vi "StartAll.vi"(8 "Error In":errorcluster[](array[cluster])) -> (0 "Error Out":errorcluster[](array[cluster]), 2 "BC_AppInfo":T1)   [LabVIEW 2014, in "BusController.lvlib"]
uses:
  BusController.lvlib
  Modules/AppModule/PublicAPI/Arguments/Requests/BC_AppInfo.ctl
  Admin/Registry/BCReg.lvclass
  Queue/QueueType.ctl
  Admin/BCAdmin.lvclass/BCAdmin.ctl
  Admin/Accessors/Read BCRegRef.vi
  BusController.vi
  Bus_class/Bus.lvclass
  Framework.lvlib
  <userlib>/NIST/NISTErrorLib/NISTErrorLib.lvlib
  Modules/AppModule/AppModule.lvlib
  Admin/BCAdmin.lvclass
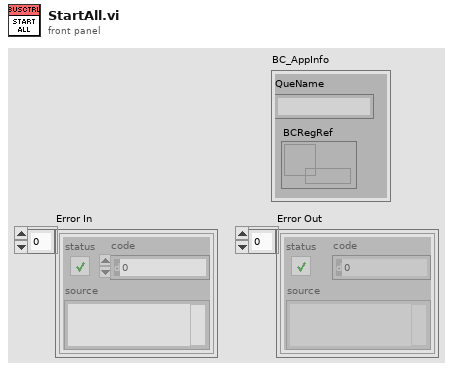
[diagram p1: front panel]
types:
  T1 = typedef "AppModule.lvlib/BC_AppInfo.ctl" = cluster{"QueName":string, "BCRegRef":refnum<data-value>}
  T2 = typedef "BusController.lvlib/QueueType.ctl" = cluster{"Msg":string, "Data":variant}
  T3 = typedef "Framework.lvlib/clFrameworkData.ctl" = cluster{"EvtINIFilePaths":path[], "BusClassInstances":refnum<class "Bus.lvclass">[], "PmuImpairINIFilePaths":path[], "FlagImpairINIFilePaths":path[], "NetImpairINIFilePaths":path[], "OutputToFileINIFilePaths":path[], "AppINIFilePaths":path[], "AppModuleID":i32, "OutputToFileID":i32}
  T4 = typedef "Rendezvous RefNum" = refnum<k1>
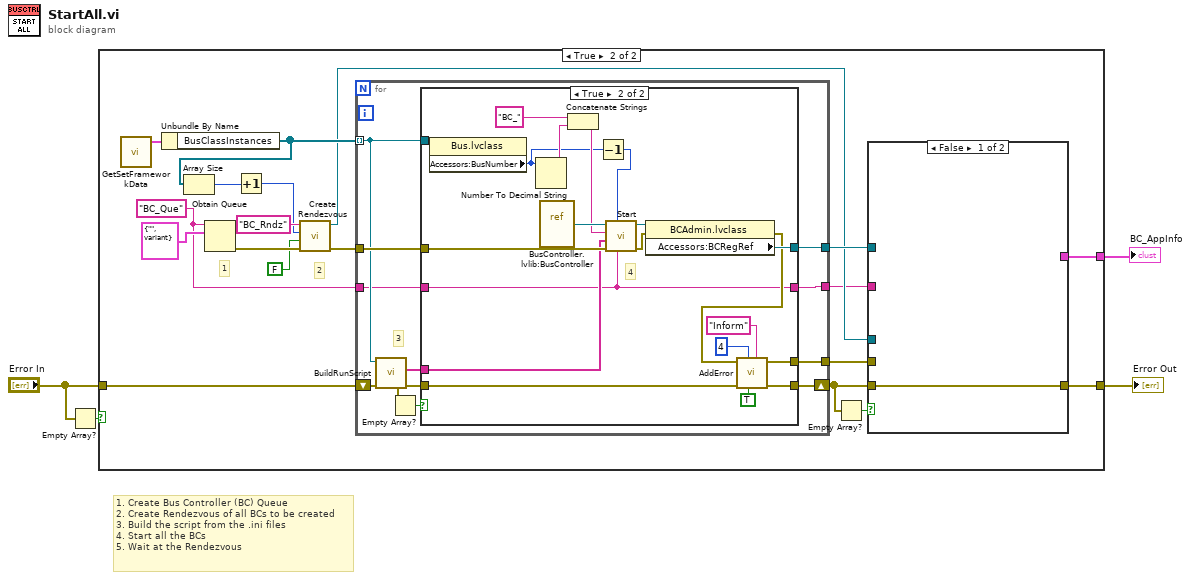
[diagram p0: block diagram]
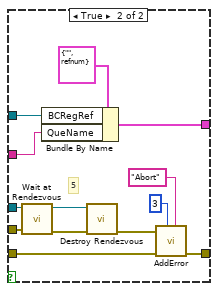
[diagram p3: hidden frame]
diagram:
  # "1. Create Bus Controller (BC) Queue\n2. Create Rendezvous of all BCs to be created\n3. Build the script from the .ini files\n4. Start all the BCs\n5. Wait at the Rendezvous"
  n1 = Empty Array?(array="Error In") -> (empty?=w4:bool)
  n2 = case shown="True" w4 {
    tunnel: "Error In" -> [w5 w21]
    tunnel: [w5 w13] -> w2
    tunnel: [_ w20] -> w1
    frame False {
    }
    frame True {
      w9 = "BC_Que" ("name (unnamed)")
      # "2"
      # "1"
      n3 = call "GetSetFrameworkData.vi"() -> ("clFrameworkData Out"=w24:T3)  [unwired: 11 in]
      n4 = Unbundle By Name(w24) -> ("BusClassInstances"=w16:refnum<class "Bus.lvclass">[])
      n5 = Array Size(array=w16) -> (size(s)=w12:i32)
      n6 = Obtain Queue(name (unnamed)=w9, element data type=T2 {"Msg"="", "Data"=variant} ("QueueType")) -> (error out=w19:errorcluster)  [unwired: 3 in, 2 out]
      n7 = Increment(x=w12) -> (x+1=w11:i32)
      n8 = call <vilib>:"Create Rendezvous.vi"("error in (no error)"=w19, "return existing (F)"=FALSE, "size (2)"=w11, "name (unnamed)"="BC_Rndz") -> ("error out"=w18:errorcluster, "rendezvous"=w14:T4)  [unwired: 1 in, 1 out]
      n9 = for {
        tunnel: w16 -> [w45] mode=indexing
        tunnel: w18 -> [w49]
        tunnel: [w48] -> w22
        shift-right: [w47] -> w6
        shift-left: w21 -> [w46]
        tunnel: [w43] -> w15
        tunnel: w9 -> [w42]
        tunnel: [w41] -> w8
        # "3"
        n10 = call "BuildRunScript.vi"("ErrorArray"=w46, "Bus"=w45) -> ("ErrorArray"=w39:errorcluster[], "Script"=w44:string[])  [unwired: 7 in, 1 out]
        n11 = Empty Array?(array=w39) -> (empty?=w40:bool)
        n12 = case shown="True" w40 {
          tunnel: w49 -> [_ w66]
          tunnel: [_ w64] -> w48
          tunnel: [w50 w62] -> w47
          tunnel: w39 -> [w50 w58]
          tunnel: w45 -> [_ w57]
          tunnel: w44 -> [_ w56]
          tunnel: [_ w52] -> w43
          tunnel: w42 -> [_ w51]
          tunnel: [_ w51] -> w41
          frame False {
          }
          frame True {
            # "4"
            n13 = property class="Bus.lvclass"(reference=w57) -> ("Accessors:BusNumber"=w55:u8)  [unwired: 1 in, 2 out]
            n14 = Number To Decimal String(number=w55) -> (decimal integer string=w69:string)  [unwired: 1 in]
            n15 = vi-ref "BusController.lvlib:BusController.vi"() -> (w70:refnum<vi>)
            n16 = Concatenate Strings("BC_", w69) -> (w67:string)
            n17 = Decrement(x=w55) -> (x-1=w54:u8)
            n18 = call "Start.vi"("BcQueName"=w51, "BusIndex"=w54, "error in (no error)"=w66, "Script"=w56, "Name"=w67, "VI Refnum"=w70) -> ("error out"=w63:errorcluster, "BCAdmin"=w65:refnum<class "BCAdmin.lvclass">)  [unwired: 3 in, 1 out]
            n19 = property class="BCAdmin.lvclass"(reference=w65, error in=w63) -> (error out=w61:errorcluster, "Accessors:BCRegRef"=w64:refnum<data-value>)  [unwired: 1 out]
            n20 = call <userlib>:"AddError.vi"("Severity"="Inform", "Passthrough (f)"=TRUE, "Priority"=u8 4, "ErrorArray"=w58, "error in (no error)"=w61) -> ("ErrorArray"=w62:errorcluster[], "error out"=w52:errorcluster)  [unwired: 5 in]
          }
        }
      }
      n21 = Empty Array?(array=w6) -> (empty?=w7:bool)
      n22 = case shown="False" w7 {
        tunnel: w22 -> [_ w37]
        tunnel: [_ w36] -> w20
        tunnel: w15 -> [_ w35]
        tunnel: w14 -> [_ w34]
        tunnel: w6 -> [w25 w31]
        tunnel: [w25 w30] -> w13
        tunnel: w8 -> [_ w27]
        frame False {
        }
        frame True {
          # "5"
          n23 = call <vilib>:"Wait at Rendezvous.vi"("error in (no error)"=w35, "rendezvous"=w34) -> ("error out"=w33:errorcluster, "rendezvous out"=w32:T4)  [unwired: 3 in, 1 out]
          n24 = Bundle By Name(cluster=T1 {"QueName"="", "BCRegRef"=refnum} ("BC_AppInfo"), "BCRegRef"=w37, "QueName"=w27) -> (w36:T1)
          n25 = call <vilib>:"Destroy Rendezvous.vi"("error in (no error)"=w33, "rendezvous"=w32) -> ("error out"=w26:errorcluster)  [unwired: 4 in, 1 out]
          n26 = call <userlib>:"AddError.vi"("Severity"="Abort", "Priority"=u8 3, "ErrorArray"=w31, "error in (no error)"=w26) -> ("ErrorArray"=w30:errorcluster[])  [unwired: 6 in, 1 out]
        }
      }
    }
  }
  "Error Out" <- w2
  "BC_AppInfo" <- w1
